vi "查询上序合格Z100.vi"(8 "error in (no error)":errorcluster, 11 "产品ID":string) -> (0 "error out":errorcluster, 1 "本序已做":bool, 2 "上序合格":bool)   [LabVIEW 2011]
uses:
  <vilib>/Utility/error.llb/whitespace.ctl
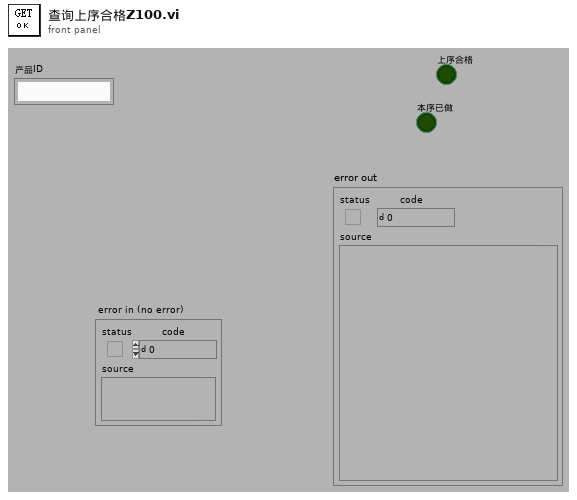
[diagram p1: front panel]
types:
  T1 = typedef "whitespace.ctl" = u16
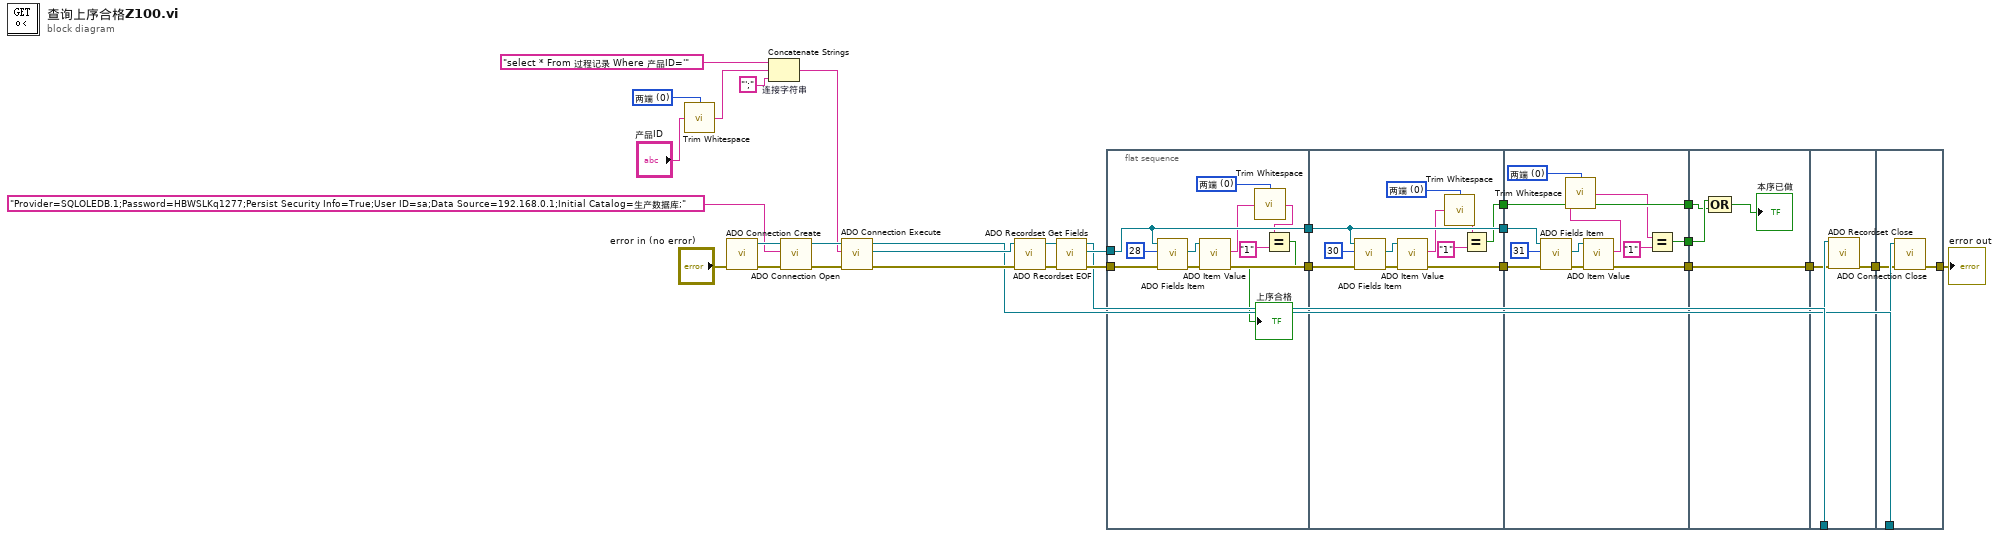
[diagram p0: block diagram]
diagram:
  w20 = T1 0 items=["两端", "字符串首端", "字符串末端"] ("location (both)")
  n1 = call <vilib>:"Trim Whitespace.vi"("string"="产品ID", "location (both)"=w20) -> ("trimmed string"=w21:string)
  n2 = call "ADO Connection Create.vi"("error in (no error)"="error in (no error)") -> ("error out"=w30:errorcluster, "ADODB._Connection Out"=w31:refnum<k7>)  [unwired: 9 out]
  n3 = Concatenate Strings "连接字符串"("select * From 过程记录 Where 产品ID='" ("字符串 2"), w21, "';" ("字符串 2")) -> (w19:string)
  n4 = call "ADO Connection Open.vi"("error in (no error)"=w30, "ConnectionString"="Provider=SQLOLEDB.1;Password=HBWSLKq1277;Persist Security Info=True;User ID=sa;Data Source=192.168.0.1;Initial Catalog=生产数据库;" ("字符串 2"), "ADODB._Connection In"=w31) -> ("error out"=w29:errorcluster, "ADODB._Connection Out"=w28:refnum<k7>)  [unwired: 7 out]
  n5 = call "ADO Connection Execute.vi"("error in (no error)"=w29, "CommandText"=w19, "ADODB._Connection In"=w28) -> ("error out"=w25:errorcluster, "RecordSet"=w26:refnum<k7>, "ADODB._Connection Out"=w11:refnum<k7>)  [unwired: 6 out]
  n6 = call "ADO Recordset EOF.vi"("error in (no error)"=w25, "ADODB._Recordset In"=w26) -> ("error out"=w16:errorcluster, "ADODB._Recordset Out"=w17:refnum<k7>)  [unwired: 8 out]
  n7 = call "ADO Recordset Get Fields.vi"("error in (no error)"=w16, "ADODB._Recordset In"=w17) -> ("error out"=w14:errorcluster, "Fields Out"=w15:refnum<k7>, "ADODB._Recordset Out"=w12:refnum<k7>)  [unwired: 7 out]
  n8 = flat-sequence {
    tunnel: w15 -> [w37]
    tunnel: w14 -> [w38]
    tunnel: [w42] -> w8
    tunnel: [w37] -> w7
    tunnel: w8 -> [w50]
    tunnel: w7 -> [w47]
    tunnel: [w49] -> w5
    tunnel: [w47] -> w4
    tunnel: [w46] -> w2
    tunnel: [w61] -> w6
    tunnel: w5 -> [w62]
    tunnel: w4 -> [w59]
    tunnel: [w58] -> w3
    tunnel: w2 -> [w57]
    tunnel: [w57] -> w1
    tunnel: w6 -> [w69]
    tunnel: [w69] -> w13
    tunnel: w3 -> [w68]
    tunnel: w1 -> [w67]
    tunnel: w13 -> [w71]
    tunnel: w12 -> [w72]
    tunnel: [w70] -> w10
    tunnel: w11 -> [w75]
    tunnel: w10 -> [w74]
    tunnel: [w73] -> w9
    frame #0 {
      w35 = T1 0 items=["两端", "字符串首端", "字符串末端"] ("location (both)")
      n9 = call "ADO Fields Item.vi"("error in (no error)"=w38, "Index"=28, "Fields In"=w37) -> ("error out"=w40:errorcluster, "Item Out"=w39:refnum<k7>)  [unwired: 7 out]
      n10 = call "ADO Item Value.vi"("error in (no error)"=w40, "Item In"=w39) -> ("error out"=w42:errorcluster, "Value"=w34:string)  [unwired: 8 out]
      n11 = call <vilib>:"Trim Whitespace.vi"("string"=w34, "location (both)"=w35) -> ("trimmed string"=w33:string)
      n12 = Equal?(x=w33, y="1") -> (x = y?=→"上序合格":bool)
    }
    frame #1 {
      w45 = T1 0 items=["两端", "字符串首端", "字符串末端"] ("location (both)")
      n13 = call "ADO Fields Item.vi"("error in (no error)"=w50, "Index"=30, "Fields In"=w47) -> ("error out"=w52:errorcluster, "Item Out"=w51:refnum<k7>)  [unwired: 7 out]
      n14 = call "ADO Item Value.vi"("error in (no error)"=w52, "Item In"=w51) -> ("error out"=w49:errorcluster, "Value"=w44:string)  [unwired: 8 out]
      n15 = call <vilib>:"Trim Whitespace.vi"("string"=w44, "location (both)"=w45) -> ("trimmed string"=w43:string)
      n16 = Equal?(x=w43, y="1") -> (x = y?=w46:bool)
    }
    frame #2 {
      w56 = T1 0 items=["两端", "字符串首端", "字符串末端"] ("location (both)")
      n17 = call "ADO Fields Item.vi"("error in (no error)"=w62, "Index"=31, "Fields In"=w59) -> ("error out"=w64:errorcluster, "Item Out"=w63:refnum<k7>)  [unwired: 7 out]
      n18 = call "ADO Item Value.vi"("error in (no error)"=w64, "Item In"=w63) -> ("error out"=w61:errorcluster, "Value"=w55:string)  [unwired: 8 out]
      n19 = call <vilib>:"Trim Whitespace.vi"("string"=w55, "location (both)"=w56) -> ("trimmed string"=w54:string)
      n20 = Equal?(x=w54, y="1") -> (x = y?=w58:bool)
    }
    frame #3 {
      n21 = Compound Arithmetic op=OR(w68, w67) -> (→"本序已做":bool)
    }
    frame #4 {
      n22 = call "ADO Recordset Close.vi"("ADODB._Recordset In"=w72, "error in (no error)"=w71) -> ("error out"=w70:errorcluster)  [unwired: 17 out]
    }
    frame #5 {
      n23 = call "ADO Connection Close.vi"("error in (no error)"=w74, "ADODB._Connection In"=w75) -> ("error out"=w73:errorcluster)  [unwired: 9 out]
    }
  }
  "error out" <- w9
